vi "Equip-Set active.vi"(0 "Listbox ref":refnum<vi>, 2 "Save to file?":bool, 11 "error in (no error)":errorcluster) -> (15 "error out":errorcluster)   [LabVIEW 2015]
uses:
  <vilib>/Utility/config.llb/Write Key (String).vi
  <vilib>/Utility/config.llb/NI_LVConfig.lvlib
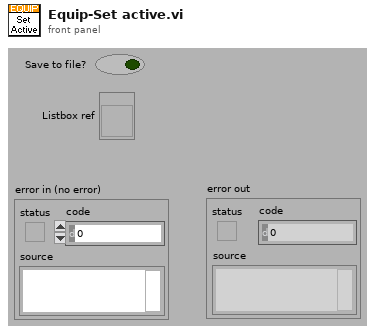
[diagram p1: front panel]
types:
  T1 = typedef "NI_LVConfig.lvlib/Config Data RefNum.ctl" = refnum<k1>
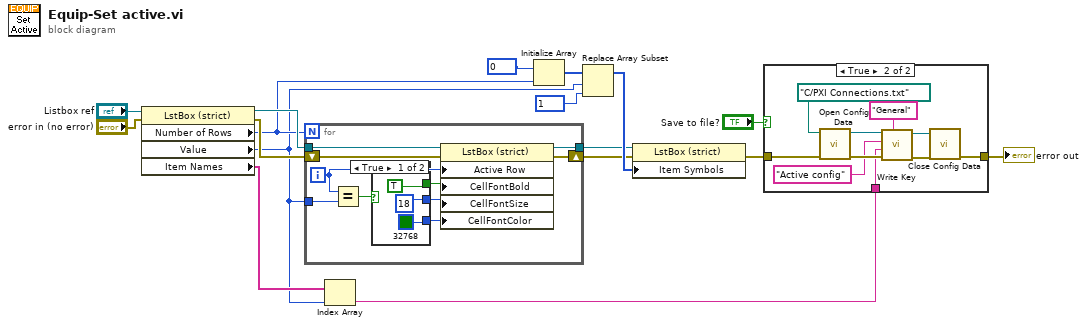
[diagram p0: block diagram]
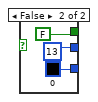
[diagram p3: hidden frame]
diagram:
  n1 = property class="LstBox (strict)"(reference="Listbox ref", error in="error in (no error)") -> (reference out=w15:refnum<vi>, error out=w16:errorcluster, "Number of Rows"=w14:u32, "Value"=w3:i32, "Item Names"=w4:string[])
  n2 = for {
    N: w14 -> [_]
    tunnel: w15 -> [w23]
    shift-right: [w25] -> w8
    shift-left: w16 -> [w24]
    tunnel: w3 -> [w21]
    tunnel: [w18] -> w7
    i -> [w20]
    n3 = Equal?(x=w20, y=w21) -> (x = y?=w22:bool)
    n4 = case shown="True" w22 {
      tunnel: [TRUE ("Active Row:Cell Font:Bold") FALSE ("Active Row:Cell Font:Bold")] -> w27
      tunnel: [u32 18 ("Active Row:Cell Font:Size") u32 13 ("Active Row:Cell Font:Size")] -> w26
      tunnel: [u32 32768 u32 0] -> w19
      frame True {
      }
      frame False {
      }
    }
    n5 = property class="LstBox (strict)"(reference=w23, error in=w24, "Active Row"=w20, "CellFontBold"=w27, "CellFontSize"=w26, "CellFontColor"=w19) -> (reference out=w18:refnum<vi>, error out=w25:errorcluster)
  }
  n6 = Index Array(array=w4, index=w3) -> (element=w2:string)
  n7 = Initialize Array(0, w14) -> (w11:i32[])
  n8 = Replace Array Subset(array=w11, new element=1, index=w3) -> (w9:i32[])
  n9 = property class="LstBox (strict)"(reference=w7, error in=w8, "Item Symbols"=w9) -> (error out=w6:errorcluster)  [unwired: 1 out]
  n10 = case shown="True" "Save to file?" {
    tunnel: w6 -> [w34 w44]
    tunnel: [w34 w39] -> w5
    tunnel: w2 -> [_ w36]
    frame False {
    }
    frame True {
      n11 = call <vilib>:"Open Config Data.vi"("error in (no error)"=w44, "configuration file path"=path "C:/PXI Connections.txt") -> ("error out"=w43:errorcluster, "refnum"=w42:T1)  [unwired: 7 in, 1 out]
      n12 = call-poly <vilib>:"Write Key.vi"("section"="General", "error in (no error)"=w43, "value"=w36, "key"="Active config", "refnum"=w42) -> ("error out"=w41:errorcluster, "refnum out"=w40:T1)  [unwired: 4 in, 1 out]
      n13 = call <vilib>:"Close Config Data.vi"("error in (no error)"=w41, "refnum"=w40) -> ("error out"=w39:errorcluster)  [unwired: 8 in, 1 out]
    }
  }
  "error out" <- w5
